vi "Utility - Configuration File Generator.vi"() -> ()   [LabVIEW 2014]
uses:
  controls/Master Configuration.ctl
  controls/EPICS Configuration.ctl
  <vilib>/Utility/xml.llb/Write to XML File(string).vi
panel:
  in  "Master Configuration":T1={"Epics Configuration"={"DIN Mask"=[], "# Samples Post Trig"=300000, "Armed"=FALSE, "ADC Mask"=[], "ADC Max Threshold"=[], "ADC Min Threshold"=[]}, "Epics Configuration File"="c:\\EpicsConfig.cfg", "Number of Channels"=16, "Data rate"=0, "PM Buffer Size"=0}
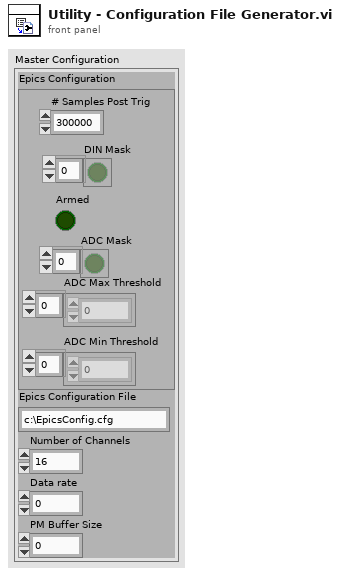
[diagram p1: front panel]
types:
  T1 = typedef "Master Configuration.ctl" = cluster{"Epics Configuration":T2, "Epics Configuration File":string, "Number of Channels":u8, "Data rate":u32, "PM Buffer Size":u32}
  T2 = typedef "EPICS Configuration.ctl" = cluster{"DIN Mask":bool[], "# Samples Post Trig":u32, "Armed":bool, "ADC Mask":bool[], "ADC Max Threshold":dbl[], "ADC Min Threshold":dbl[]}
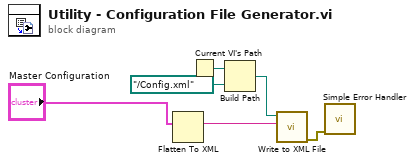
[diagram p0: block diagram]
diagram:
  n1 = Flatten To XML(anything="Master Configuration") -> (xml string=w6:string)
  n2 = Current VI's Path() -> (path=w5:path)
  n3 = Build Path(base path=w5, name or relative path=path "../Config.xml") -> (appended path=w3:path)
  n4 = call-poly <vilib>:"Write to XML File.vi"("XML Input"=w6, "XML File Path"=w3) -> ("error out"=w2:errorcluster)  [unwired: 7 in, 2 out]
  n5 = call <vilib>:"Simple Error Handler.vi"("error in (no error)"=w2) -> ()  [unwired: 4 in, 5 out]
